vi "fgv_vlp16_databuf.vi"(7 "cmd":T2, 8 "error in":errorcluster, 10 "xyz_data":cluster{"x":dbl, "y":dbl, "z":dbl}[](array[cluster]), 11 "raw data in":T1(array[cluster])=array[29568 elements]) -> (0 "error out":errorcluster, 2 "xyz_data_out":cluster{"x":dbl, "y":dbl, "z":dbl}[](array[cluster]), 3 "raw data out":T1(array[cluster]))   [LabVIEW 2019]
uses:
  Ctrl/vlp-16 cmd.ctl
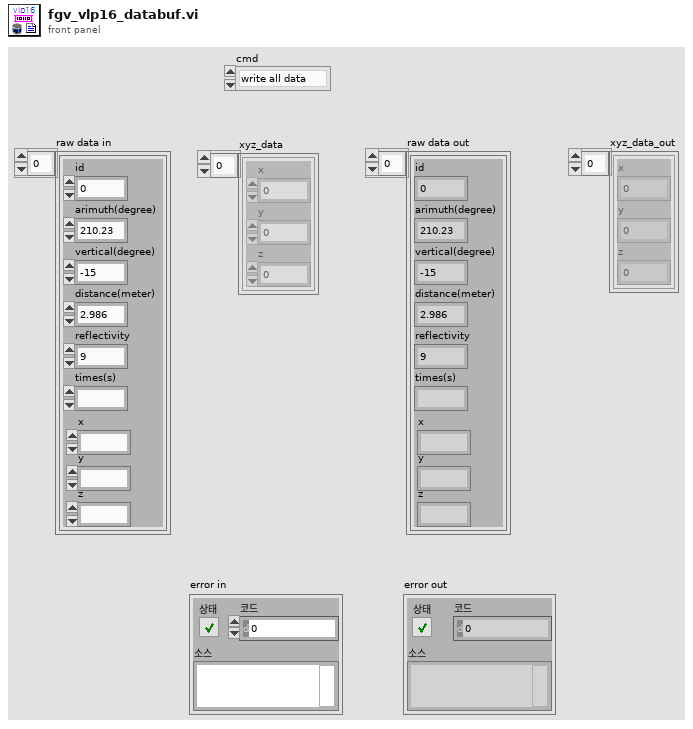
[diagram p1: front panel]
types:
  T1 = cluster{"id":i32, "arimuth(degree)":dbl, "vertical(degree)":dbl, "distance(meter)":dbl, "reflectivity":u8, "times(s)":ext, "x":dbl, "y":dbl, "z":dbl}[]
  T2 = typedef "vlp-16 cmd.ctl" = enum16{"write all data", "write xyz data", "read"}
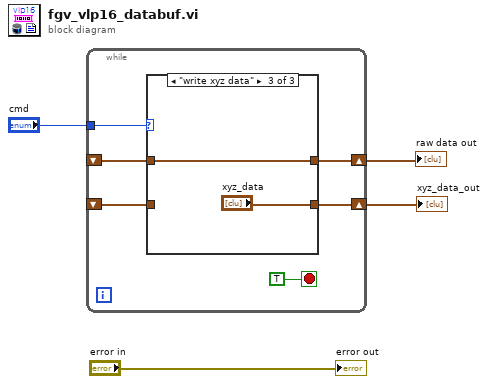
[diagram p0: block diagram]
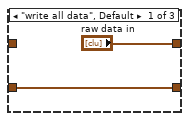
[diagram p2: hidden frame]
diagram:
  n1 = while {
    tunnel: "cmd" -> [w9]
    shift-right: [w8] -> w3
    shift-left: _ -> [w7]
    shift-right: [w6] -> w1
    shift-left: _ -> [w5]
    stop <- TRUE stop-if-true
    n2 = case shown="\"write xyz data\"" w9 {
      tunnel: ["raw data in" w14 w16] -> w8
      tunnel: w7 -> [_ w14 w16]
      tunnel: [w11 w13 "xyz_data"] -> w6
      tunnel: w5 -> [w11 w13 _]
      frame "write all data", Default {
      }
      frame "read" {
      }
      frame "write xyz data" {
      }
    }
  }
  "raw data out" <- w3
  "xyz_data_out" <- w1
  "error out" <- "error in"
